vi "Arithmetic.vi"() -> ()   [LabVIEW 2019]
panel:
  out "x+y":dbl
  in  "Numeric 2":dbl
  in  "Numeric 1":dbl
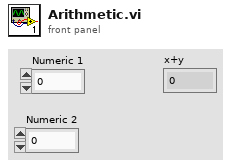
[diagram p1: front panel]
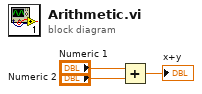
[diagram p0: block diagram]
diagram:
  n1 = Add(x="Numeric 1", y="Numeric 2") -> (x+y=→"x+y":dbl)
